vi "Detect MSw.vi"(9 "Side Gyro Data":T2={"Time"=0.0, "Gyro Array Data"=[], "Gyro Negation"=[], "Gyro Data"={"Gyro X"=0.0, "Gyro Y"=0.0, "Gyro Z"=0.0}, "Gyro Latency"=0.0, "Normalization Time"=640.0, "Sampling Rate"=0.0}, 10 "Side Event Data":T1={"Event Data"={"LR"={"Phase"="LR", "On"=FALSE, "Last On Time"=0.0, "Duration"=0.0, "Crossing Time"=0.0, "Time since LR"=0.0, "Time Since TSw"=0.0, "Min gyro Z"=0.0, "Time since LR?"=FALSE, "Time since TSw?"=FALSE, "Min gyro Z?"=FALSE, "Crossing?"=FALSE}, "MSt"={"Phase"="MSt", "On"=FALSE, "Last On Time"=0.0, "Duration"=0.0}, "TSt"={"Phase"="TSt", "On"=FALSE, "Last On Time"=0.0, "Duration"=0.0}, "PSw"={"Phase"="PSw", "On"=FALSE, "Last On Time"=0.0, "Duration"=0.0}, "ISw"={"Phase"="ISw", "On"=FALSE, "Last On Time"=0.0, "Duration"=0.0, "Peak Time"=0.0, "Time since LR"=0.0, "Time since ISw"=0.0, "Time since LR?"=FALSE, "Time since ISw?"=FALSE, "Peak?"=FALSE}, "MSw"={"Phase"="MSw", "On"=FALSE, "Last On Time"=0.0, "Duration"=0.0, "Crossing time"=0.0, "Time since LR"=0.0, "Time since MSw"=0.0, "Time since ISw"=0.0, "Time since LR?"=FALSE, "Time since MSw?"=FALSE, "Time since ISw?"=FALSE, "Crossing?"=FALSE}, "TSw"={"Phase"="TSw", "On"=FALSE, "Last On Time"=0.0, "Duration"=0.0, "Peak time"=0.0, "Time since LR"=0.0, "Time since TSw"=0.0, "Time since LR?"=FALSE, "Time since TSw?"=FALSE, "Peak?"=FALSE}}, "Mean Cycle Duration"=0.0, "Event Detected?"=FALSE, "Last Event Detected"=0, "Num Cycles"=0.0, "GPD Log"=refnum, "Last Event Time"=0.0}, 11 "GPD Parameters":T4={"% Cycle Delay"=0.0, "Min % Cycle LR to ISw "=0.0, "Min % Cycle LR to MSw"=0.0, "Min % Cycle LR to TSw"=0.0, "Max % Cycle ISw to MSw"=0.0, "Min % Cycle TSw to LR"=0.0, "Max % Cycle TSw to LR"=0.0, "LR Min Gyro Z Threshold"=0.0, "LR Min Gyro Z Width"=0.0, "ISw Peak Threshold"=0.0, "ISw Peak Width"=0.0, "TSw Valley Threshold"=0.0, "TSw Valley Width (ms)"=7.0, "Max Cycle Time (s)"=0.0, "Mean Computation Window"=0.0, "CP subject?"=FALSE}) -> (1 "Gyro Data Out":T2={"Time"=0.0, "Gyro Array Data"=[], "Gyro Negation"=[], "Gyro Data"={"Gyro X"=0.0, "Gyro Y"=0.0, "Gyro Z"=0.0}, "Gyro Latency"=0.0, "Normalization Time"=640.0, "Sampling Rate"=0.0}, 2 "Side Event Data":T1={"Event Data"={"LR"={"Phase"="LR", "On"=FALSE, "Last On Time"=0.0, "Duration"=0.0, "Crossing Time"=0.0, "Time since LR"=0.0, "Time Since TSw"=0.0, "Min gyro Z"=0.0, "Time since LR?"=FALSE, "Time since TSw?"=FALSE, "Min gyro Z?"=FALSE, "Crossing?"=FALSE}, "MSt"={"Phase"="MSt", "On"=FALSE, "Last On Time"=0.0, "Duration"=0.0}, "TSt"={"Phase"="TSt", "On"=FALSE, "Last On Time"=0.0, "Duration"=0.0}, "PSw"={"Phase"="PSw", "On"=FALSE, "Last On Time"=0.0, "Duration"=0.0}, "ISw"={"Phase"="ISw", "On"=FALSE, "Last On Time"=0.0, "Duration"=0.0, "Peak Time"=0.0, "Time since LR"=0.0, "Time since ISw"=0.0, "Time since LR?"=FALSE, "Time since ISw?"=FALSE, "Peak?"=FALSE}, "MSw"={"Phase"="MSw", "On"=FALSE, "Last On Time"=0.0, "Duration"=0.0, "Crossing time"=0.0, "Time since LR"=0.0, "Time since MSw"=0.0, "Time since ISw"=0.0, "Time since LR?"=FALSE, "Time since MSw?"=FALSE, "Time since ISw?"=FALSE, "Crossing?"=FALSE}, "TSw"={"Phase"="TSw", "On"=FALSE, "Last On Time"=0.0, "Duration"=0.0, "Peak time"=0.0, "Time since LR"=0.0, "Time since TSw"=0.0, "Time since LR?"=FALSE, "Time since TSw?"=FALSE, "Peak?"=FALSE}}, "Mean Cycle Duration"=0.0, "Event Detected?"=FALSE, "Last Event Detected"=0, "Num Cycles"=0.0, "GPD Log"=refnum, "Last Event Time"=0.0}, 3 "GPD Parameters out":T4={"% Cycle Delay"=0.0, "Min % Cycle LR to ISw "=0.0, "Min % Cycle LR to MSw"=0.0, "Min % Cycle LR to TSw"=0.0, "Max % Cycle ISw to MSw"=0.0, "Min % Cycle TSw to LR"=0.0, "Max % Cycle TSw to LR"=0.0, "LR Min Gyro Z Threshold"=0.0, "LR Min Gyro Z Width"=0.0, "ISw Peak Threshold"=0.0, "ISw Peak Width"=0.0, "TSw Valley Threshold"=0.0, "TSw Valley Width (ms)"=7.0, "Max Cycle Time (s)"=0.0, "Mean Computation Window"=0.0, "CP subject?"=FALSE}, 4 "MSw Detected?":bool)   [LabVIEW 2019]
uses:
  Controls/Gyro Side Data.ctl
  Controls/Gyro Negation.ctl
  Controls/GPD Side Parameters.ctl
  Controls/Side Event Data.ctl
  <vilib>/ptbypt/NI_PtbyPt.lvlib
panel:
  out "x .or. y?":bool
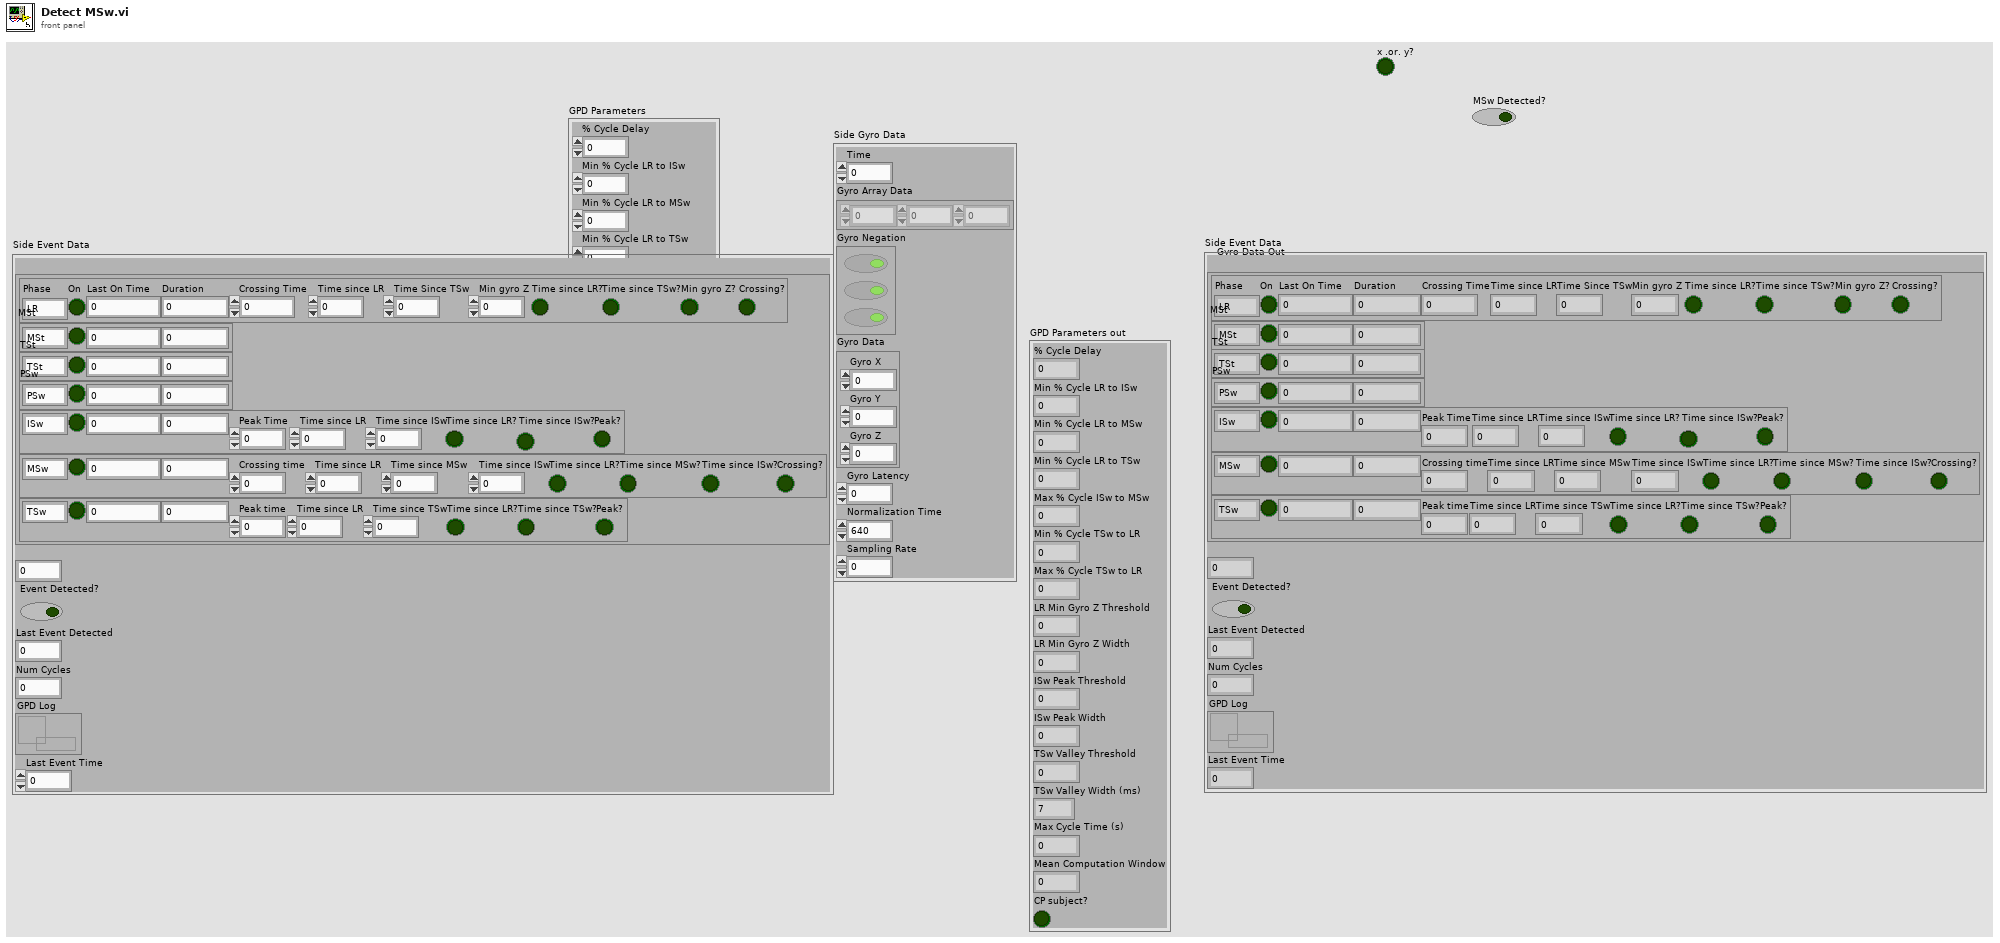
[diagram p1: front panel]
types:
  T1 = typedef "Side Event Data.ctl" = cluster{"Event Data":cluster{"LR":cluster{"Phase":string, "On":bool, "Last On Time":dbl, "Duration":dbl, "Crossing Time":dbl, "Time since LR":dbl, "Time Since TSw":dbl, "Min gyro Z":dbl, "Time since LR?":bool, "Time since TSw?":bool, "Min gyro Z?":bool, "Crossing?":bool}, "MSt":cluster{"Phase":string, "On":bool, "Last On Time":dbl, "Duration":dbl}, "TSt":cluster{"Phase":string, "On":bool, "Last On Time":dbl, "Duration":dbl}, "PSw":cluster{"Phase":string, "On":bool, "Last On Time":dbl, "Duration":dbl}, "ISw":cluster{"Phase":string, "On":bool, "Last On Time":dbl, "Duration":dbl, "Peak Time":dbl, "Time since LR":dbl, "Time since ISw":dbl, "Time since LR?":bool, "Time since ISw?":bool, "Peak?":bool}, "MSw":cluster{"Phase":string, "On":bool, "Last On Time":dbl, "Duration":dbl, "Crossing time":dbl, "Time since LR":dbl, "Time since MSw":dbl, "Time since ISw":dbl, "Time since LR?":bool, "Time since MSw?":bool, "Time since ISw?":bool, "Crossing?":bool}, "TSw":cluster{"Phase":string, "On":bool, "Last On Time":dbl, "Duration":dbl, "Peak time":dbl, "Time since LR":dbl, "Time since TSw":dbl, "Time since LR?":bool, "Time since TSw?":bool, "Peak?":bool}}, "Mean Cycle Duration":dbl, "Event Detected?":bool, "Last Event Detected":i32, "Num Cycles":dbl, "GPD Log":refnum<queue>, "Last Event Time":dbl}
  T2 = typedef "Gyro Side Data.ctl" = cluster{"Time":dbl, "Gyro Array Data":dbl[], "Gyro Negation":T3, "Gyro Data":cluster{"Gyro X":dbl, "Gyro Y":dbl, "Gyro Z":dbl}, "Gyro Latency":dbl, "Normalization Time":dbl, "Sampling Rate":dbl}
  T3 = typedef "Gyro Negation.ctl" = bool[]
  T4 = typedef "GPD Side Parameters.ctl" = cluster{"% Cycle Delay":dbl, "Min % Cycle LR to ISw ":dbl, "Min % Cycle LR to MSw":dbl, "Min % Cycle LR to TSw":dbl, "Max % Cycle ISw to MSw":dbl, "Min % Cycle TSw to LR":dbl, "Max % Cycle TSw to LR":dbl, "LR Min Gyro Z Threshold":dbl, "LR Min Gyro Z Width":dbl, "ISw Peak Threshold":dbl, "ISw Peak Width":dbl, "TSw Valley Threshold":dbl, "TSw Valley Width (ms)":dbl, "Max Cycle Time (s)":dbl, "Mean Computation Window":dbl, "CP subject?":bool}
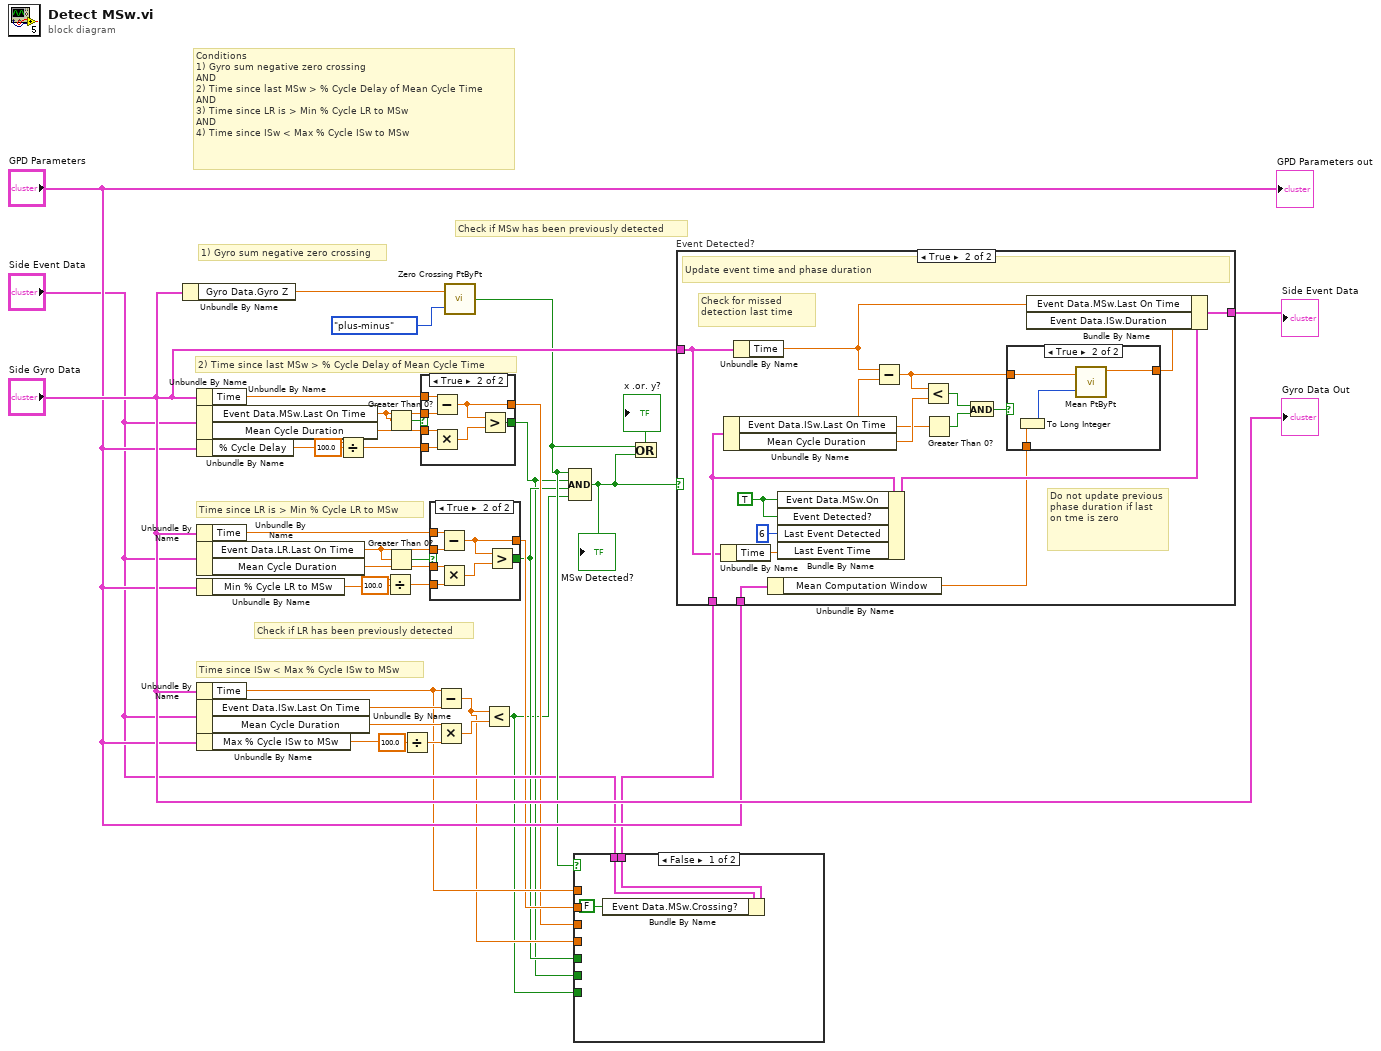
[diagram p0: block diagram]
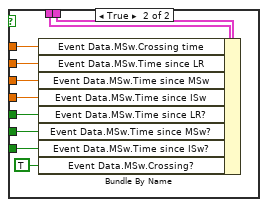
[diagram p2: hidden frame]
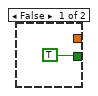
[diagram p3: hidden frame]
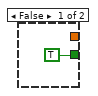
[diagram p4: hidden frame]
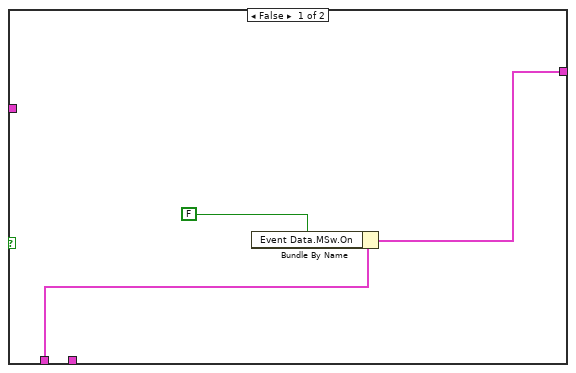
[diagram p5: hidden frame]
diagram:
  # "Check if LR has been previously detected"
  # "Check if MSw has been previously detected"
  # "Time since ISw < Max % Cycle ISw to MSw"
  # "Time since LR is > Min % Cycle LR to MSw"
  # "2) Time since last MSw > % Cycle Delay of Mean Cycle Time"
  # "1) Gyro sum negative zero crossing"
  # "Conditions\n1) Gyro sum negative zero crossing\nAND\n2) Time since last MSw > % Cycle Delay of Mean Cycle Time\nAND\n3) Time since LR is > Min % Cycle LR to MSw\nAND\n4) Time since ISw < Max % Cycle ISw to MSw"
  n1 = Unbundle By Name("Side Gyro Data") -> ("Gyro Data.Gyro Z"=w17:dbl)
  n2 = Unbundle By Name("Side Gyro Data") -> ("Time"=w24:dbl)
  n3 = Unbundle By Name("Side Event Data") -> ("Event Data.MSw.Last On Time"=w14:dbl, "Mean Cycle Duration"=w23:dbl)
  n4 = Unbundle By Name("GPD Parameters") -> ("% Cycle Delay"=w35:dbl)
  n5 = Unbundle By Name("Side Gyro Data") -> ("Time"=w30:dbl)
  n6 = Unbundle By Name("Side Event Data") -> ("Event Data.LR.Last On Time"=w12:dbl, "Mean Cycle Duration"=w31:dbl)
  n7 = Unbundle By Name("GPD Parameters") -> ("Min % Cycle LR to MSw"=w32:dbl)
  n8 = Unbundle By Name("Side Gyro Data") -> ("Time"=w7:dbl)
  n9 = Unbundle By Name("Side Event Data") -> ("Event Data.ISw.Last On Time"=w20:dbl, "Mean Cycle Duration"=w29:dbl)
  n10 = Unbundle By Name("GPD Parameters") -> ("Max % Cycle ISw to MSw"=w27:dbl)
  n11 = Divide(x=w35, y=100.0) -> (x/y=w22:dbl)
  n12 = Divide(x=w32, y=100.0) -> (x/y=w21:dbl)
  n13 = Greater Than 0?(x=w14) -> (x > 0?=w11:bool)
  n14 = Greater Than 0?(x=w12) -> (x > 0?=w13:bool)
  n15 = Divide(x=w27, y=100.0) -> (x/y=w19:dbl)
  n16 = case shown="True" w11 {
    tunnel: w24 -> [_ w45]
    tunnel: w14 -> [_ w44]
    tunnel: w23 -> [_ w43]
    tunnel: w22 -> [_ w42]
    tunnel: [TRUE w40] -> w2
    tunnel: [_ w39] -> w5
    frame False {
    }
    frame True {
      n17 = Subtract(x=w45, y=w44) -> (x-y=w39:dbl)
      n18 = Multiply(x=w43, y=w42) -> (x*y=w41:dbl)
      n19 = Greater?(x=w39, y=w41) -> (0:w40:bool)
    }
  }
  n20 = case shown="True" w13 {
    tunnel: w31 -> [_ w53]
    tunnel: w30 -> [_ w52]
    tunnel: w12 -> [_ w51]
    tunnel: w21 -> [_ w50]
    tunnel: [TRUE w48] -> w3
    tunnel: [_ w47] -> w6
    frame False {
    }
    frame True {
      n21 = Subtract(x=w52, y=w51) -> (x-y=w47:dbl)
      n22 = Multiply(x=w53, y=w50) -> (x*y=w49:dbl)
      n23 = Greater?(x=w47, y=w49) -> (0:w48:bool)
    }
  }
  n24 = Subtract(x=w7, y=w20) -> (x-y=w4:dbl)
  n25 = Multiply(x=w29, y=w19) -> (x*y=w18:dbl)
  n26 = call <vilib>:"Zero Crossing PtByPt.vi"("direction"=enum16{"either", "minus-plus", "plus-minus"}."plus-minus", "input data point"=w17) -> ("crossing"=w10:bool)  [unwired: 1 in]
  n27 = Less?(x=w4, y=w18) -> (x < y?=w1:bool)
  n28 = Compound Arithmetic op=AND(w10, w2, w3, w1) -> (w16:bool)
  "MSw Detected?" <- w16
  n29 = case shown="False" w10 {
    tunnel: "Side Event Data" -> [w56 w66]
    tunnel: [w55 w65] -> w8
    tunnel: w7 -> [_ w64]
    tunnel: w6 -> [_ w63]
    tunnel: w5 -> [_ w62]
    tunnel: w4 -> [_ w61]
    tunnel: w3 -> [_ w60]
    tunnel: w2 -> [_ w59]
    tunnel: w1 -> [_ w58]
    frame False {
      n30 = Bundle By Name(cluster=w56, "Event Data.MSw.Crossing?"=FALSE) -> (w55:T1)
    }
    frame True {
      n31 = Bundle By Name(cluster=w66, "Event Data.MSw.Crossing time"=w64, "Event Data.MSw.Time since LR"=w63, "Event Data.MSw.Time since MSw"=w62, "Event Data.MSw.Time since ISw"=w61, "Event Data.MSw.Time since LR?"=w60, "Event Data.MSw.Time since MSw?"=w59, "Event Data.MSw.Time since ISw?"=w58, "Event Data.MSw.Crossing?"=TRUE) -> (w65:T1)
    }
  }
  n32 = Or(x=w10, y=w16) -> (x .or. y?=→"x .or. y?":bool)
  n33 = case "Event Detected?" shown="True" w16 {
    tunnel: w8 -> [w68 w82]
    tunnel: [w67 w86] -> w37
    tunnel: "Side Gyro Data" -> [_ w70]
    tunnel: "GPD Parameters" -> [_ w77]
    frame False {
      n34 = Bundle By Name(cluster=w68, "Event Data.MSw.On"=FALSE) -> (w67:T1)
    }
    frame True {
      w79 = TRUE
      # "Do not update previous phase duration if last on tme is zero"
      # "Check for missed detection last time"
      # "Update event time and phase duration"
      n35 = Unbundle By Name(w70) -> ("Time"=w71:dbl)
      n36 = Unbundle By Name(w82) -> ("Event Data.ISw.Last On Time"=w72:dbl, "Mean Cycle Duration"=w85:dbl)
      n37 = Unbundle By Name(w70) -> ("Time"=w80:dbl)
      n38 = Unbundle By Name(w77) -> ("Mean Computation Window"=w76:dbl)
      n39 = Bundle By Name(cluster=w82, "Event Data.MSw.On"=w79, "Event Detected?"=w79, "Last Event Detected"=6, "Last Event Time"=w71) -> (w81:T1)
      n40 = Subtract(x=w80, y=w72) -> (x-y=w84:dbl)
      n41 = Less?(x=w84, y=w85) -> (x < y?=w74:bool)
      n42 = Greater Than 0?(x=w72) -> (x > 0?=w75:bool)
      n43 = And(x=w74, y=w75) -> (x .and. y?=w73:bool)
      n44 = case shown="True" w73 {
        tunnel: w84 -> [w87 w91]
        tunnel: [w87 w90] -> w83
        tunnel: w76 -> [_ w89]
        frame False {
        }
        frame True {
          n45 = To Long Integer(number=w89) -> (32bit integer=w88:i32)
          n46 = call <vilib>:"Mean PtByPt.vi"("x"=w91, "sample length"=w88) -> ("mean"=w90:dbl)  [unwired: 2 in, 1 out]
        }
      }
      n47 = Bundle By Name(cluster=w81, "Event Data.MSw.Last On Time"=w80, "Event Data.ISw.Duration"=w83) -> (w86:T1)
    }
  }
  "Side Event Data" <- w37
  "GPD Parameters out" <- "GPD Parameters"
  "Gyro Data Out" <- "Side Gyro Data"
